vi "Sum trees.vi"(8 "len":i32, 9 "start":i32, 10 "Add_to_tree[]":T1(array[cluster]), 11 "TreeItems[]":T1(array[cluster])) -> (3 "Tree_Out[]":T1(array[cluster]))   [LabVIEW 2021, in "Tree.lvlib" / "Tree.lvclass"]
uses:
  Tree.lvclass
  Tree.lvclass/Tree.ctl
panel:
  # "Процедура \"сложения\" деревьев.\nДонор Add_to_tree отдает свой элемент в Tree"
  # "Add_to_tree"
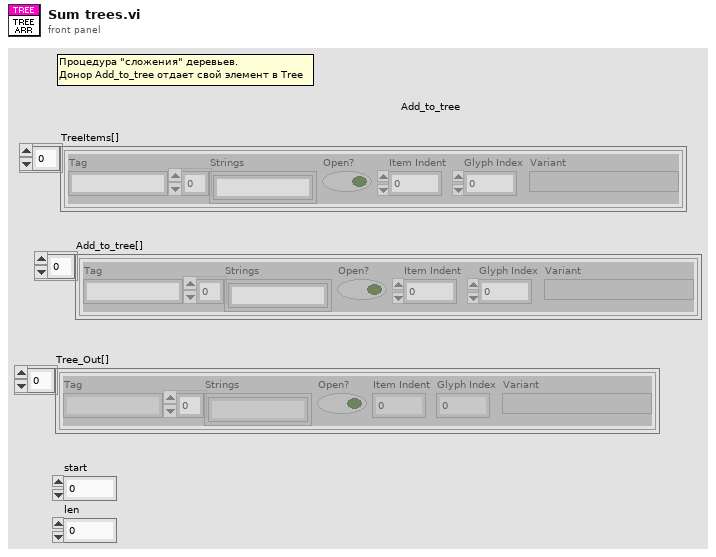
[diagram p1: front panel]
types:
  T1 = cluster{"Tag":string, "Strings":string[], "Open?":bool, "Item Indent":i32, "Glyph Index":i32, "Variant":variant}[]
  T2 = cluster{"Tag":string, "Strings":string[], "Open?":bool, "Item Indent":i32, "Glyph Index":i32, "Variant":variant}
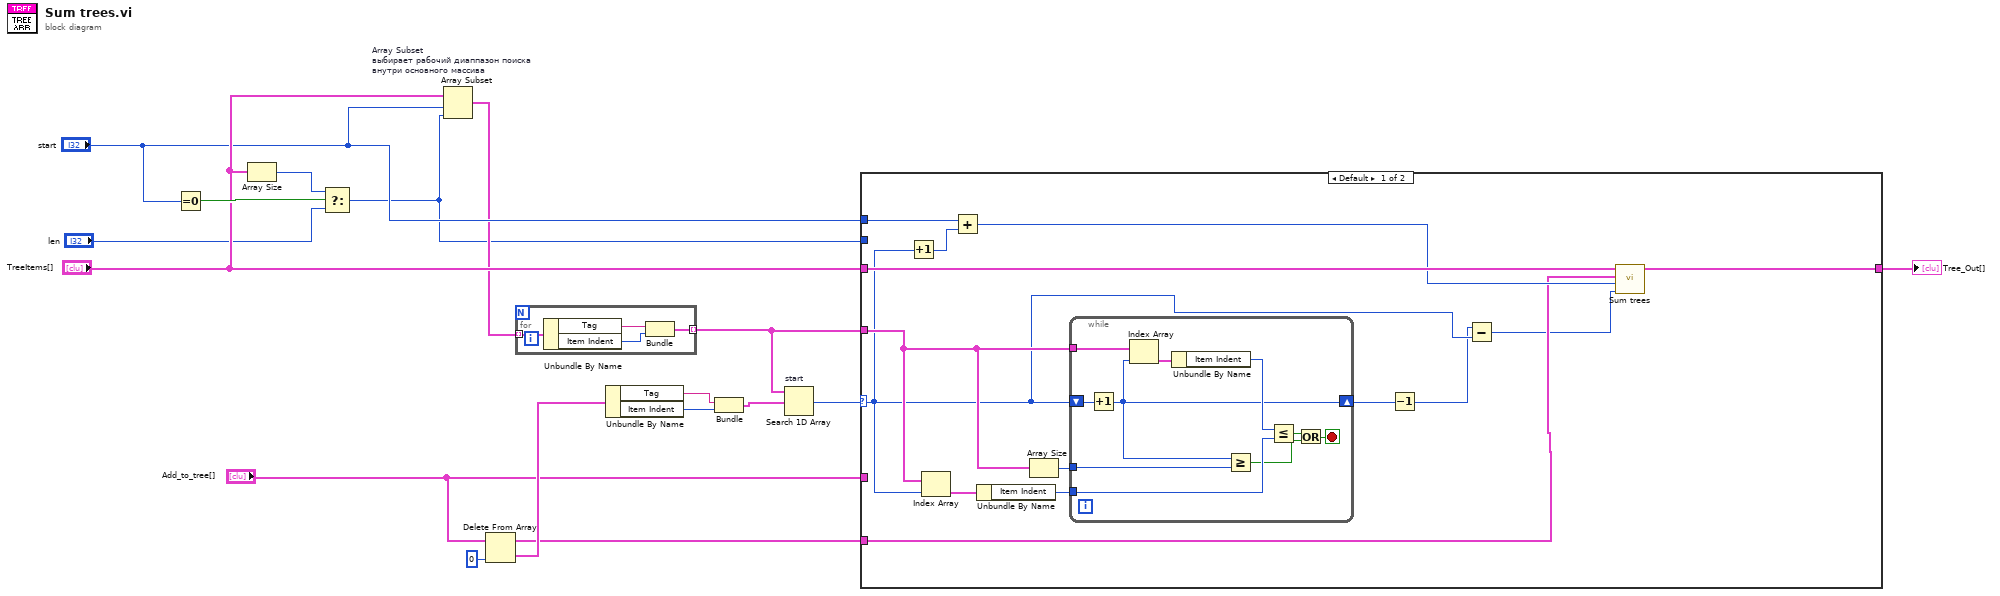
[diagram p0: block diagram]
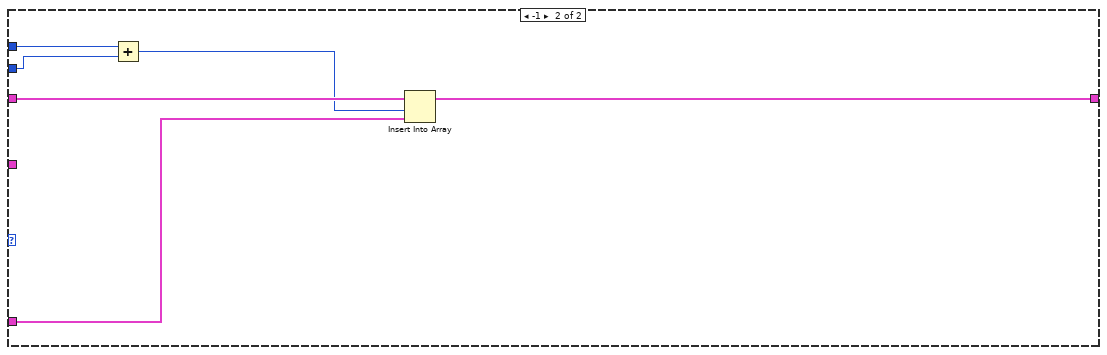
[diagram p2: hidden frame]
diagram:
  n1 = Equal To 0?(x="start") -> (x = 0?=w8:bool)
  n2 = Array Size(array="TreeItems[]") -> (size(s)=w7:i32)
  n3 = Select(t=w7, s=w8, f="len") -> (s? t:f=w2:i32)
  n4 = Array Subset "Array Subset\nвыбирает рабочий диаппазон поиска\nвнутри основного массива"(array="TreeItems[]", index="start", length=w2) -> (w3:T1)
  n5 = Delete From Array(array="Add_to_tree[]", index=0) -> (deleted portion=w11:T2, array with subset deleted=w10:T1)  [unwired: 1 in]
  n6 = for {
    tunnel: w3 -> [w21] mode=indexing
    tunnel: [w19] -> w17 mode=indexing
    n7 = Unbundle By Name(w21) -> ("Tag"=w20:string, "Item Indent"=w18:i32)
    n8 = Bundle("Tag"=w20, "Item Indent"=w18) -> (w19:cluster{"Tag":string, "Item Indent":i32})  [unwired: 1 in]
  }
  n9 = Unbundle By Name(w11) -> ("Tag"=w14:string, "Item Indent"=w12:i32)
  n10 = Bundle("Tag"=w14, "Item Indent"=w12) -> (w13:cluster{"Tag":string, "Item Indent":i32})  [unwired: 1 in]
  n11 = Search 1D Array "start"(1D array=w17, element=w13) -> (index of element=w6:i32)  [unwired: 1 in]
  n12 = case shown="Default" w6 {
    selector: w6 -> [w24 _]
    tunnel: [w34 w51] -> w16
    tunnel: "TreeItems[]" -> [w35 w48]
    tunnel: w17 -> [w31 _]
    tunnel: w10 -> [w26 _]
    tunnel: "Add_to_tree[]" -> [_ w46]
    tunnel: "start" -> [w29 w50]
    tunnel: w2 -> [_ w49]
    frame Default {
      n13 = Increment(x=w24) -> (x+1=w27:i32)
      n14 = Index Array(array=w31, index=w24) -> (element=w33:cluster{"Tag":string, "Item Indent":i32})
      n15 = Add(x=w29, y=w27) -> (x+y=w28:i32)
      n16 = Unbundle By Name(w33) -> ("Item Indent"=w32:i32)
      n17 = Array Size(array=w31) -> (size(s)=w30:i32)
      n18 = while {
        tunnel: w31 -> [w45]
        shift-right: [w38] -> w25
        shift-left: w24 -> [w44]
        tunnel: w32 -> [w41]
        tunnel: w30 -> [w39]
        stop <- w37 stop-if-true
        n19 = Increment(x=w44) -> (x+1=w38:i32)
        n20 = Index Array(array=w45, index=w38) -> (element=w43:cluster{"Tag":string, "Item Indent":i32})
        n21 = Unbundle By Name(w43) -> ("Item Indent"=w42:i32)
        n22 = Greater Or Equal?(x=w38, y=w39) -> (x >= y?=w36:bool)
        n23 = Less Or Equal?(x=w42, y=w41) -> (x <= y?=w40:bool)
        n24 = Or(x=w40, y=w36) -> (x .or. y?=w37:bool)
      }
      n25 = Decrement(x=w25) -> (x-1=w22:i32)
      n26 = Subtract(x=w22, y=w24) -> (x-y=w23:i32)
      n27 = call "Sum trees.vi"("len"=w23, "start"=w28, "Add_to_tree[]"=w26, "TreeItems[]"=w35) -> ("Tree_Out[]"=w34:T1)  [unwired: 7 in]
    }
    frame -1 {
      n28 = Add(x=w50, y=w49) -> (x+y=w47:i32)
      n29 = Insert Into Array(array=w48, index=w47, new element=w46) -> (w51:T1)
    }
  }
  "Tree_Out[]" <- w16
